vi "ex6-7.vi"   [LabVIEW 2013]
uses:
  <vilib>/NXT/Dual Mode Library/Waits/Wait_Rotation.vi
  <vilib>/NXT/Dual Mode Library/Display/drawNumber.vi
  <vilib>/NXT/NXTIO Xnodes/NXTIONodeSubVIs/LEGOMoveAllMotors.vi
  <vilib>/NXT/Subs/LVHSConnector.ctl
  <vilib>/NXT/NXTIO Xnodes/NXTIOXNode/NXTIO.xnode
  <vilib>/NXT/LegoClasses/BrickReference/BrickReference.lvclass
types:
  T1 = typedef "LVHSConnector.ctl" = refnum<class "BrickReference.lvclass">
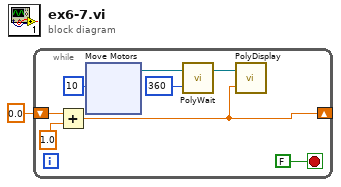
[diagram p0: block diagram]
diagram:
  n1 = while {
    shift-right: [w3] -> _
    shift-left: 0.0 -> [w2]
    stop <- FALSE stop-if-true
    n2 = Add(x=w2, y=1.0) -> (x+y=w3:dbl)
    n3 = xnode "Move Motors"("Power/Speed 1"=i8 10) -> ("NXT/EV3"=w7:T1)  [unwired: 2 in]
    n4 = call-poly <vilib>:"PolyWait.vi"("Position Change (180)"=360, "NXT/EV3"=w7) -> ("NXT/EV3"=w6:T1)  [unwired: 2 in]
    n5 = call-poly <vilib>:"PolyDisplay.vi"("number"=w3, "NXT/EV3"=w6) -> ()  [unwired: 2 in, 1 out]
  }
